vi "LWXPS_ZygoErrorStatusGet.vi"(0 "XPS Reference IN":refnum<k24>, 5 "Axis":i32, 11 "LabVIEW error IN":errorcluster) -> (4 "XPS Reference OUT":refnum<k24>, 6 "Returned error code":i32, 8 "Error status":string, 10 "XPS Error String":string, 15 "LabVIEW error OUT":errorcluster)   [LabVIEW 2014]
uses:
  D:/XPSQ8_LabView_Library/Development/Source/Dll/Newport.XPS.CommandInterface.dll
  Dll/Newport.XPS.CommandInterface.dll
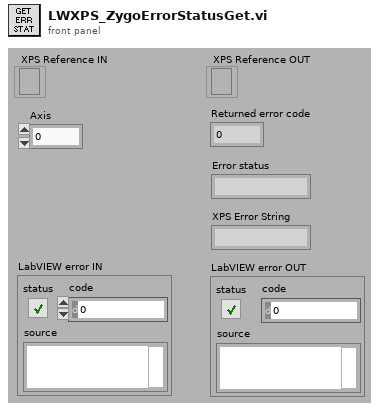
[diagram p1: front panel]
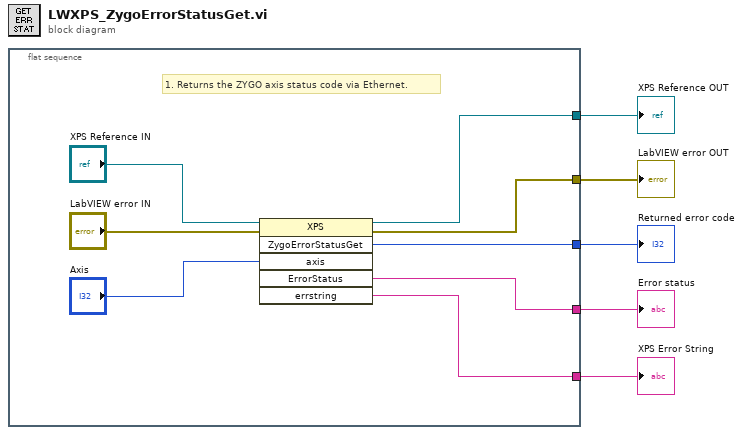
[diagram p0: block diagram]
diagram:
  n1 = flat-sequence {
    tunnel: [w11] -> w5
    tunnel: [w9] -> w4
    tunnel: [w12] -> w3
    tunnel: [w7] -> w2
    tunnel: [w6] -> w1
    frame #0 {
      # "1. Returns the ZYGO axis status code via Ethernet."
      n2 = invoke class="XPS" method="ZygoErrorStatusGet"(reference="XPS Reference IN", error in="LabVIEW error IN", "axis"="Axis") -> (reference out=w11:refnum<k24>, error out=w9:errorcluster, "ZygoErrorStatusGet"=w12:i32, "ErrorStatus"=w7:string, "errstring"=w6:string)  [unwired: 3 in, 1 out]
    }
  }
  "XPS Error String" <- w1
  "XPS Reference OUT" <- w5
  "LabVIEW error OUT" <- w4
  "Returned error code" <- w3
  "Error status" <- w2
